vi "FF+FB control.vi"() -> ()   [LabVIEW 2010]
uses:
  <vilib>/DAQmx/read.llb/DAQmx Read (Analog 1D DBL NChan 1Samp).vi
  <vilib>/DAQmx/write.llb/DAQmx Write (Analog DBL 1Chan 1Samp).vi
  <vilib>/DAQmx/create/channels.llb/DAQmx Create Channel (AI-Voltage-Basic).vi
  <vilib>/DAQmx/configure/timing.llb/DAQmx Timing (Sample Clock).vi
  <vilib>/DAQmx/create/channels.llb/DAQmx Create Channel (AO-Voltage-Basic).vi
  <vilib>/daqmx/miscellaneous.llb/DAQmx Fill In Error Info.vi
panel:
  in  "ch2 Kii 增益":dbl=-10000.0
  in  "ch1 Kii 增益":dbl=-10000.0
  in  "ch2 Kp 增益":dbl=0.13
  out "overload":bool
  in  "ch1 Kp 增益":dbl=-250.0
  in  "ch2 Ki 增益":dbl=83.5
  in  "ch1 Ki 增益":dbl=-10000.0
  in  "估測DC時間(秒) 2":dbl=2.0
  in  "估測DC時間(秒) 3":dbl=1.0
  out "Waveform Chart 16":dbl(graph)=0.004379241651609749
  out "Waveform Chart 15":dbl(graph)=0.009421818236378054
  out "Waveform Chart 14":dbl(graph)=7.749143729656655e-05
  out "Waveform Chart 13":dbl(graph)=-2.8609948748865505e-06
  in  "Controller on":bool
  out "error out":errorcluster
  out "Waveform Chart 10":dbl(graph)=-0.0027164247368556514
  out "Waveform Chart 9":dbl(graph)=0.00014048287990779042
  out "延遲百分比(%)  需小於0.5%":dbl=2.0072842804614854
  out "理想迴圈時間(ms)":dbl=0.11111111111111112
  out "迴圈平均運行時間(ms)":dbl=0.11334142697829055
  in  "output channels 1":tag="PXI-6733/ao0"
  in  "stop":bool
  in  "估測DC時間(秒) 1":dbl=2.0
  in  "每通道取樣頻率(Hz)":dbl=9000.0 format="%0.2f"
  in  "input channels 2":tag="PXI-6229/ai1"
  in  "input channels 1":tag="PXI-6229/ai0"
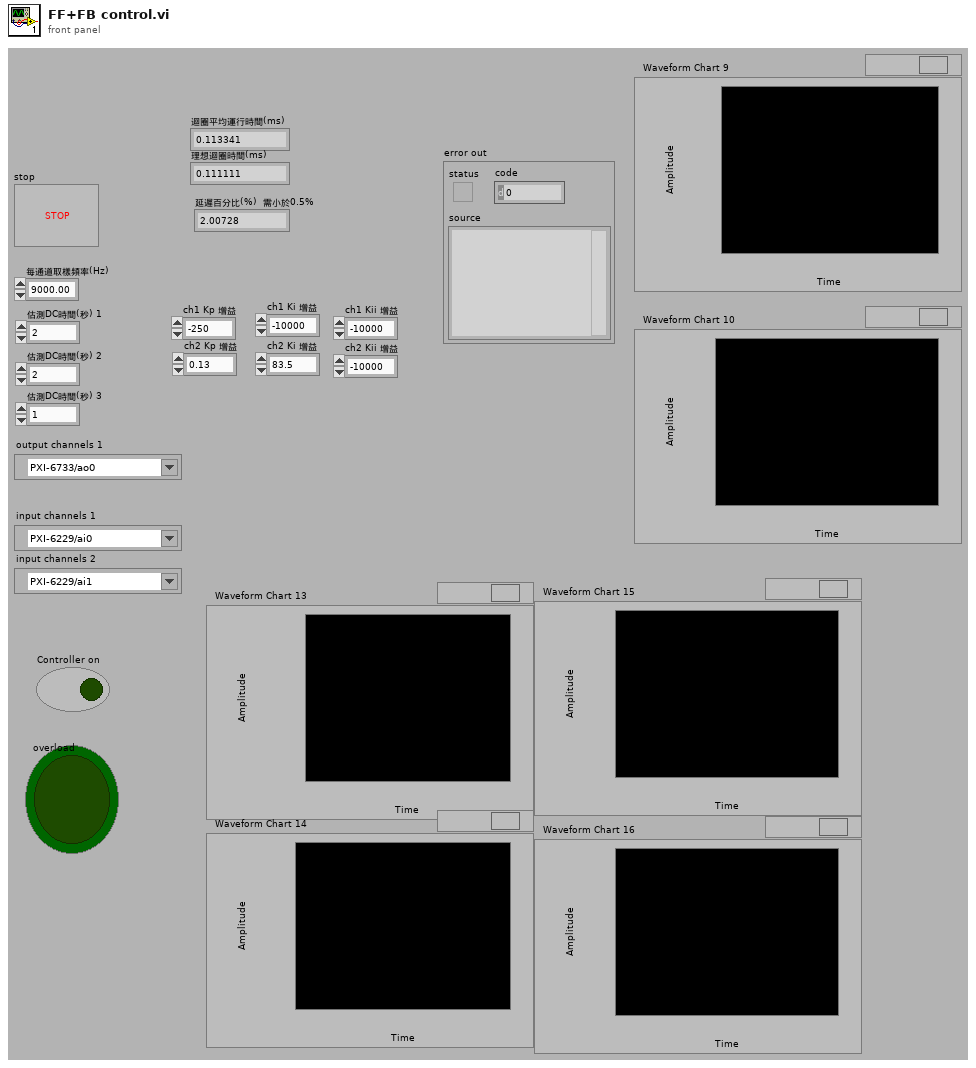
[diagram p1: front panel]
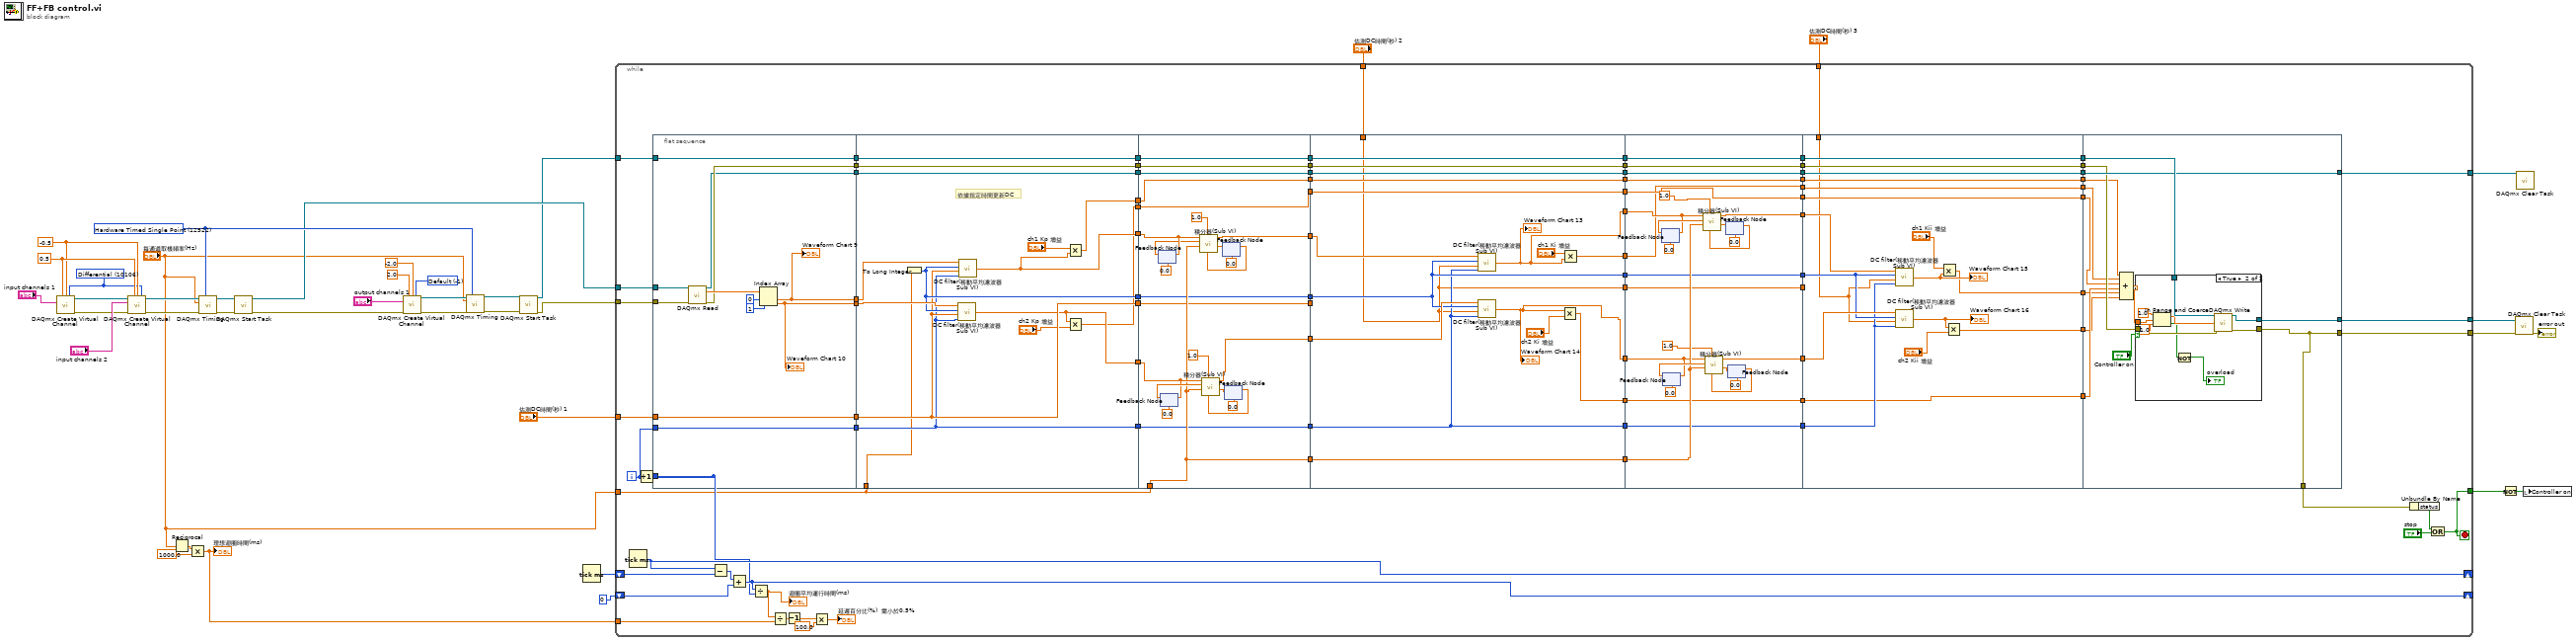
[diagram p0: block diagram]
diagram:
  w26 = -1 items=["Default"=-1, "RSE"=10083, "Differential"=10106, "Pseudodifferential"=12529] ("output terminal configuration")
  w23 = 12522 items=["Finite Samples"=10178, "Continuous Samples"=10123, "Hardware Timed Single Point"=12522] ("sample mode")
  w34 = 10106 items=["default"=-1, "RSE"=10083, "NRSE"=10078, "Differential"=10106, "Pseudodifferential"=12529] ("input terminal configuration")
  w35 = -0.5 ("minimum value")
  w36 = 0.5 ("maximum value")
  n1 = call-poly <vilib>:"DAQmx Create Virtual Channel.vi"("maximum value"=w36, "minimum value"=w35, "input terminal configuration"=w34, "physical channels"="input channels 1") -> ("task out"=w39:refnum<k21>, "error out"=w31:errorcluster)  [unwired: 10 in]
  n2 = call-poly <vilib>:"DAQmx Create Virtual Channel.vi"("task in"=w39, "maximum value"=w36, "minimum value"=w35, "input terminal configuration"=w34, "physical channels"="input channels 2", "error in"=w31) -> ("task out"=w33:refnum<k21>, "error out"=w30:errorcluster)  [unwired: 8 in]
  n3 = Reciprocal(x="每通道取樣頻率(Hz)") -> (1/x=w14:dbl)
  n4 = Multiply(x=w14, y=1000.0) -> (x*y=w12:dbl)
  "理想迴圈時間(ms)" <- w12
  n5 = call-poly <vilib>:"DAQmx Timing.vi"("task/channels in"=w33, "sample mode"=w23, "rate"="每通道取樣頻率(Hz)", "error in"=w30) -> ("task out"=w32:refnum<k21>, "error out"=w29:errorcluster)  [unwired: 10 in]
  n6 = call <vilib>:"DAQmx Start Task.vi"("task/channels in"=w32, "error in"=w29) -> ("task out"=w19:refnum<k21>, "error out"=w20:errorcluster)  [unwired: 12 in]
  n7 = call-poly <vilib>:"DAQmx Create Virtual Channel.vi"("maximum value"=2.0, "minimum value"=-2.0 ("maximum value"), "output terminal configuration"=w26, "physical channels"="output channels 1", "error in"=w20) -> ("task out"=w25:refnum<k21>, "error out"=w24:errorcluster)  [unwired: 9 in]
  n8 = call-poly <vilib>:"DAQmx Timing.vi"("task/channels in"=w25, "sample mode"=w23, "rate"="每通道取樣頻率(Hz)", "error in"=w24) -> ("task out"=w22:refnum<k21>, "error out"=w21:errorcluster)  [unwired: 10 in]
  n9 = call <vilib>:"DAQmx Start Task.vi"("task/channels in"=w22, "error in"=w21) -> ("task out"=w10:refnum<k21>, "error out"=w18:errorcluster)  [unwired: 12 in]
  n10 = Tick Count (ms)() -> (millisecond timer value=w16:u32)
  n11 = while {
    tunnel: w19 -> [w128]
    tunnel: w18 -> [w127]
    shift-right: [w123] -> _
    shift-left: w16 -> [w124]
    shift-right: [w120] -> _
    shift-left: 0 ("index") -> [w121]
    tunnel: w12 -> [w117]
    tunnel: "每通道取樣頻率(Hz)" -> [w66]
    tunnel: w10 -> [w103]
    tunnel: [w96] -> w7
    tunnel: [w64] -> w6
    tunnel: [w83] -> w5
    tunnel: "估測DC時間(秒) 1" -> [w82]
    tunnel: [w65] -> w3
    tunnel: "估測DC時間(秒) 2" -> [w41]
    tunnel: "估測DC時間(秒) 3" -> [w40]
    i -> [w80]
    stop <- w65 stop-if-true
    n12 = Tick Count (ms)() -> (millisecond timer value=w123:u32)
    n13 = Increment(x=w80) -> (x+1=w119:i32)
    n14 = flat-sequence {
      tunnel: w128 -> [w140]
      tunnel: w127 -> [w139]
      tunnel: [w135] -> w126
      tunnel: [w134] -> w125
      tunnel: w119 -> [_]
      tunnel: w103 -> [w133]
      tunnel: [w133] -> w97
      tunnel: [w132] -> w95
      tunnel: [w131] -> w89
      tunnel: w82 -> [w130]
      tunnel: [w130] -> w81
      tunnel: w80 -> [w129]
      tunnel: [w129] -> w79
      tunnel: w126 -> [w152]
      tunnel: w125 -> [w151]
      tunnel: [w142] -> w112
      tunnel: [w145] -> w111
      tunnel: [w155] -> w98
      tunnel: w97 -> [w155]
      tunnel: w95 -> [w154]
      tunnel: [w154] -> w94
      tunnel: w89 -> [w153]
      tunnel: [w153] -> w84
      tunnel: w81 -> [w149]
      tunnel: w79 -> [w148]
      tunnel: [w150] -> w77
      tunnel: [w149] -> w76
      tunnel: [w148] -> w73
      tunnel: w66 -> [w147]
      tunnel: [w144] -> w56
      tunnel: [w141] -> w51
      tunnel: w112 -> [w169]
      tunnel: w111 -> [w180]
      tunnel: w66 -> [w166]
      tunnel: [w168] -> w110
      tunnel: [w167] -> w109
      tunnel: [w166] -> w106
      tunnel: [w165] -> w99
      tunnel: w98 -> [w165]
      tunnel: w94 -> [w164]
      tunnel: [w164] -> w92
      tunnel: [w163] -> w85
      tunnel: w84 -> [w163]
      tunnel: [w162] -> w78
      tunnel: w77 -> [w162]
      tunnel: w76 -> [w161]
      tunnel: [w161] -> w75
      tunnel: [w160] -> w74
      tunnel: w73 -> [w160]
      tunnel: w56 -> [w157]
      tunnel: [w157] -> w52
      tunnel: w51 -> [w156]
      tunnel: [w156] -> w50
      tunnel: w110 -> [w193]
      tunnel: w109 -> [w192]
      tunnel: [w185] -> w108
      tunnel: [w197] -> w107
      tunnel: w106 -> [w197]
      tunnel: [w196] -> w100
      tunnel: w99 -> [w196]
      tunnel: [w195] -> w93
      tunnel: w92 -> [w195]
      tunnel: [w194] -> w86
      tunnel: w85 -> [w194]
      tunnel: w78 -> [w191]
      tunnel: w75 -> [_]
      tunnel: w74 -> [w190]
      tunnel: [w191] -> w71
      tunnel: [w181] -> w69
      tunnel: [w190] -> w67
      tunnel: [w187] -> w53
      tunnel: w52 -> [w187]
      tunnel: w50 -> [w186]
      tunnel: [w186] -> w47
      tunnel: [w184] -> w44
      tunnel: [w183] -> w43
      tunnel: [w182] -> w42
      tunnel: w41 -> [w181]
      tunnel: w108 -> [w202]
      tunnel: w107 -> [w214]
      tunnel: [w213] -> w105
      tunnel: [w212] -> w104
      tunnel: [w211] -> w101
      tunnel: w100 -> [w211]
      tunnel: w93 -> [w210]
      tunnel: [w210] -> w90
      tunnel: [w209] -> w87
      tunnel: w86 -> [w209]
      tunnel: [w208] -> w72
      tunnel: w71 -> [w208]
      tunnel: [w207] -> w70
      tunnel: w69 -> [w207]
      tunnel: [w206] -> w68
      tunnel: w67 -> [w206]
      tunnel: [w198] -> w60
      tunnel: [w199] -> w57
      tunnel: [w201] -> w54
      tunnel: w53 -> [w201]
      tunnel: [w200] -> w48
      tunnel: w47 -> [w200]
      tunnel: w44 -> [w199]
      tunnel: w43 -> [w198]
      tunnel: w42 -> [w203]
      tunnel: w105 -> [w239]
      tunnel: w104 -> [w238]
      tunnel: [w242] -> w102
      tunnel: w101 -> [w242]
      tunnel: [w241] -> w91
      tunnel: w90 -> [w241]
      tunnel: [w240] -> w88
      tunnel: w87 -> [w240]
      tunnel: w72 -> [w237]
      tunnel: w70 -> [_]
      tunnel: w68 -> [w236]
      tunnel: w60 -> [w235]
      tunnel: [w235] -> w59
      tunnel: [w234] -> w58
      tunnel: w57 -> [w234]
      tunnel: [w233] -> w55
      tunnel: w54 -> [w233]
      tunnel: [w232] -> w49
      tunnel: w48 -> [w232]
      tunnel: [w227] -> w46
      tunnel: [w226] -> w45
      tunnel: w40 -> [w225]
      tunnel: w102 -> [w255]
      tunnel: [w254] -> w96
      tunnel: w91 -> [w251]
      tunnel: [w250] -> w64
      tunnel: [w253] -> w83
      tunnel: w88 -> [w253]
      tunnel: [w250] -> w63
      tunnel: w59 -> [w247]
      tunnel: w58 -> [w246]
      tunnel: w55 -> [w248]
      tunnel: w49 -> [w245]
      tunnel: w46 -> [w244]
      tunnel: w45 -> [w243]
      frame #0 {
        n15 = call-poly <vilib>:"DAQmx Read.vi"("task/channels in"=w140, "error in"=w139) -> ("task out"=w131:refnum<k21>, "data"=w136:dbl[], "error out"=w132:errorcluster)  [unwired: 11 in]
        n16 = Index Array(array=w136, index #1=0 ("index"), index #2=1 ("index")) -> (element #1=w135:dbl, element #2=w134:dbl)
        "Waveform Chart 9" <- w135
        "Waveform Chart 10" <- w134
      }
      frame #1 {
        # "依據指定時間更新DC"
        n17 = To Long Integer(number=w147) -> (32bit integer=w150:i32)
        n18 = call "DC filter(移動平均濾波器 Sub VI).vi"("當前迴圈計數(i)"=w148, "平均時間"=w149, "取樣頻率(Hz)"=w150, "input signal"=w151) -> ("DC filter output"=w142:dbl)
        n19 = call "DC filter(移動平均濾波器 Sub VI).vi"("當前迴圈計數(i)"=w148, "平均時間"=w149, "取樣頻率(Hz)"=w150, "input signal"=w152) -> ("DC filter output"=w145:dbl)
        n20 = Multiply(x="ch1 Kp 增益", y=w145) -> (x*y=w144:dbl)
        n21 = Multiply(x=w142, y="ch2 Kp 增益") -> (x*y=w141:dbl)
      }
      frame #2 {
        n22 = feedback #1(0.0) -> (w179:dbl)
        n23 = feedback-in #1(w180) -> ()
        n24 = feedback #2(0.0) -> (w170:dbl)
        n25 = feedback-in #2(w169) -> ()
        n26 = feedback #3(0.0 ("輸出累加ERR回朔")) -> (w177:dbl)
        n27 = call "積分器(Sub VI).vi"("輸入累加ERR回朔"=w177, "I增益"=1.0, "samples (Hz)"=w166, "前一個ERR"=w179, "當下ERR"=w180) -> ("輸出累加ERR回朔"=w178:dbl, "積分修正量"=w168:dbl)  [unwired: 5 in]
        n28 = feedback-in #3(w178) -> ()
        n29 = feedback #4(0.0 ("輸出累加ERR回朔")) -> (w172:dbl)
        n30 = call "積分器(Sub VI).vi"("輸入累加ERR回朔"=w172, "I增益"=1.0, "samples (Hz)"=w166, "前一個ERR"=w170, "當下ERR"=w169) -> ("輸出累加ERR回朔"=w171:dbl, "積分修正量"=w167:dbl)  [unwired: 5 in]
        n31 = feedback-in #4(w171) -> ()
      }
      frame #3 {
        n32 = call "DC filter(移動平均濾波器 Sub VI).vi"("當前迴圈計數(i)"=w190, "平均時間"=w181, "取樣頻率(Hz)"=w191, "input signal"=w193) -> ("DC filter output"=w182:dbl)
        "Waveform Chart 13" <- w182
        n33 = call "DC filter(移動平均濾波器 Sub VI).vi"("當前迴圈計數(i)"=w190, "平均時間"=w181, "取樣頻率(Hz)"=w191, "input signal"=w192) -> ("DC filter output"=w185:dbl)
        "Waveform Chart 14" <- w185
        n34 = Multiply(x=w185, y="ch2 Ki 增益") -> (x*y=w184:dbl)
        n35 = Multiply(x="ch1 Ki 增益", y=w182) -> (x*y=w183:dbl)
      }
      frame #4 {
        n36 = feedback #5(0.0) -> (w224:dbl)
        n37 = feedback-in #5(w203) -> ()
        n38 = feedback #6(0.0) -> (w215:dbl)
        n39 = feedback-in #6(w202) -> ()
        n40 = feedback #7(0.0 ("輸出累加ERR回朔")) -> (w222:dbl)
        n41 = call "積分器(Sub VI).vi"("輸入累加ERR回朔"=w222, "I增益"=1.0, "samples (Hz)"=w214, "前一個ERR"=w224, "當下ERR"=w203) -> ("輸出累加ERR回朔"=w223:dbl, "積分修正量"=w213:dbl)  [unwired: 5 in]
        n42 = feedback-in #7(w223) -> ()
        n43 = feedback #8(0.0 ("輸出累加ERR回朔")) -> (w217:dbl)
        n44 = call "積分器(Sub VI).vi"("輸入累加ERR回朔"=w217, "I增益"=1.0, "samples (Hz)"=w214, "前一個ERR"=w215, "當下ERR"=w202) -> ("輸出累加ERR回朔"=w216:dbl, "積分修正量"=w212:dbl)  [unwired: 5 in]
        n45 = feedback-in #8(w216) -> ()
      }
      frame #5 {
        n46 = call "DC filter(移動平均濾波器 Sub VI).vi"("當前迴圈計數(i)"=w236, "平均時間"=w225, "取樣頻率(Hz)"=w237, "input signal"=w239) -> ("DC filter output"=w229:dbl)
        "Waveform Chart 15" <- w229
        n47 = call "DC filter(移動平均濾波器 Sub VI).vi"("當前迴圈計數(i)"=w236, "平均時間"=w225, "取樣頻率(Hz)"=w237, "input signal"=w238) -> ("DC filter output"=w231:dbl)
        "Waveform Chart 16" <- w231
        n48 = Multiply(x="ch1 Kii 增益", y=w229) -> (x*y=w227:dbl)
        n49 = Multiply(x=w231, y="ch2 Kii 增益") -> (x*y=w226:dbl)
      }
      frame #6 {
        n50 = Compound Arithmetic op=ADD(w248, w247, w245, w246, w244, w243) -> (w249:dbl)
        n51 = case shown="True" "Controller on" {
          tunnel: w255 -> [_ w265]
          tunnel: [_ w264] -> w254
          tunnel: w251 -> [_ w263]
          tunnel: [_ w262] -> w250
          tunnel: w249 -> [_ w261]
          frame False {
          }
          frame True {
            n52 = In Range and Coerce(upper limit=1.0, x=w261, lower limit=-1.0) -> (coerced(x)=w260:dbl, In Range?=w257:bool)
            n53 = Not(x=w257) -> (.not. x?=→"overload":bool)
            n54 = call-poly <vilib>:"DAQmx Write.vi"("task/channels in"=w265, "data"=w260, "error in"=w263) -> ("task out"=w264:refnum<k21>, "error out"=w262:errorcluster)  [unwired: 10 in, 1 out]
          }
        }
      }
    }
    n55 = Subtract(x=w123, y=w124) -> (x-y=w122:u32)
    n56 = Add(x=w122, y=w121) -> (x+y=w120:u32)
    n57 = Divide(x=w120, y=w119) -> (x/y=w118:dbl)
    "迴圈平均運行時間(ms)" <- w118
    n58 = Divide(x=w118, y=w117) -> (x/y=w116:dbl)
    n59 = Decrement(x=w116) -> (x-1=w115:dbl)
    n60 = Multiply(x=w115, y=100.0) -> (x*y=→"延遲百分比(%)  需小於0.5%":dbl)
    n61 = Unbundle By Name(w63) -> ("status"=w62:bool)
    n62 = Or(x=w62, y="stop") -> (x .or. y?=w65:bool)
  }
  n63 = Not(x=w3) -> (.not. x?=w4:bool)
  n64 = call <vilib>:"DAQmx Clear Task.vi"("task in"=w7, "error in"=w6) -> ("error out"=→"error out":errorcluster)  [unwired: 13 in]
  n65 = call <vilib>:"DAQmx Clear Task.vi"("task in"=w5) -> ()  [unwired: 14 in, 1 out]
  n66 = local write "Controller on"(w4) -> ()
